vi "test_SessionManagerWrapper_StopSessionManagementService_WrapperMethodsWorkWithoutError.vi"(8 "error in":errorcluster) -> (0 "error out":errorcluster, 2 "result":string, 3 "pass":bool)   [LabVIEW 2020, in "MeasurementServerTests.lvlib" / "Session Reservation Tests.lvlib"]
uses:
  Session Reservation Tests.lvlib
  Runtime/Measurements/Measurement Plugin Session Management V1/Session Reservation/Session Reservation.lvclass
  gRPC/Generated APIs/ni/measurementlink/sessionmanagement/v1/RPC Messages/ni_measurementlink_PinMapContext.ctl
  gRPC/Generated APIs/ni/measurementlink/sessionmanagement/v1/ni.measurementlink.sessionmanagement.v1.lvlib
  gRPC/Generated APIs/ni/measurementlink/sessionmanagement/v1/RPC Messages/ni_measurementlink_sessionmanagement_v1_ReserveSessionsRequest.ctl
  Helpers/Pin Map XML Strings Global.vi
  MeasurementServerTests.lvlib
  gRPC/Generated APIs/ni/measurementlink/sessionmanagement/v1/RPC Messages/ni_measurementlink_sessionmanagement_v1_ReserveAllRegisteredSessionsRequest.ctl
  gRPC/Generated APIs/ni/measurementlink/sessionmanagement/v1/RPC Messages/ni_measurementlink_sessionmanagement_v1_ChannelMapping.ctl
  gRPC/Generated APIs/ni/measurementlink/sessionmanagement/v1/RPC Messages/nidevice_grpc_Session.ctl
  gRPC/Generated APIs/ni/measurementlink/sessionmanagement/v1/RPC Messages/ni_measurementlink_sessionmanagement_v1_SessionInformation.ctl
  gRPC/Generated APIs/ni/measurementlink/sessionmanagement/v1/RPC Messages/ni_measurementlink_sessionmanagement_v1_ReserveAllRegisteredSessionsResponse.ctl
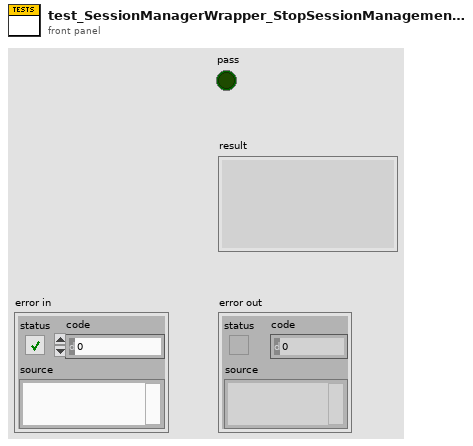
[diagram p1: front panel]
types:
  T1 = typedef "ni.measurementlink.sessionmanagement.v1.lvlib/ni_measurementlink_sessionmanagement_v1_ReserveAllRegisteredSessionsResponse.ctl" = cluster{"sessions":T2[]}
  T2 = typedef "ni.measurementlink.sessionmanagement.v1.lvlib/ni_measurementlink_sessionmanagement_v1_SessionInformation.ctl" = cluster{"session":T3, "resource_name":string, "channel_list":string, "instrument_type_id":string, "session_exists":bool, "channel_mappings":T4[]}
  T3 = typedef "ni.measurementlink.sessionmanagement.v1.lvlib/nidevice_grpc_Session.ctl" = cluster{"name":string}
  T4 = typedef "ni.measurementlink.sessionmanagement.v1.lvlib/ni_measurementlink_sessionmanagement_v1_ChannelMapping.ctl" = cluster{"pin_or_relay_name":string, "site":i32, "channel":string, "multiplexer_resource_name":string, "multiplexer_route":string}
  T5 = typedef "ni.measurementlink.sessionmanagement.v1.lvlib/ni_measurementlink_sessionmanagement_v1_ReserveAllRegisteredSessionsRequest.ctl" = cluster{"timeout_in_milliseconds":i32, "instrument_type_id":string}
  T6 = typedef "ni.measurementlink.sessionmanagement.v1.lvlib/ni_measurementlink_sessionmanagement_v1_ReserveSessionsRequest.ctl" = cluster{"pin_map_context":T7, "pin_or_relay_names":string[], "instrument_type_id":string, "timeout_in_milliseconds":i32}
  T7 = typedef "ni.measurementlink.sessionmanagement.v1.lvlib/ni_measurementlink_PinMapContext.ctl" = cluster{"pin_map_id":string, "sites":i32[]}
  T8 = typedef "ni.measurementlink.sessionmanagement.v1.lvlib/ni_measurementlink_sessionmanagement_v1_ReserveSessionsResponse.ctl" = cluster{"sessions":T2[], "multiplexer_sessions":T9[], "group_mappings":T10[]}
  T9 = typedef "ni.measurementlink.sessionmanagement.v1.lvlib/ni_measurementlink_sessionmanagement_v1_MultiplexerSessionInformation.ctl" = cluster{"session":T3, "resource_name":string, "multiplexer_type_id":string, "session_exists":bool}
  T10 = typedef "ni.measurementlink.sessionmanagement.v1.lvlib/ni_measurementlink_sessionmanagement_v1_ReserveSessionsResponse_GroupMappingsEntry.ctl" = cluster{"key":string, "value":T11}
  T11 = typedef "ni.measurementlink.sessionmanagement.v1.lvlib/ni_measurementlink_sessionmanagement_v1_ResolvedPinsOrRelays.ctl" = cluster{"pin_or_relay_names":string[]}
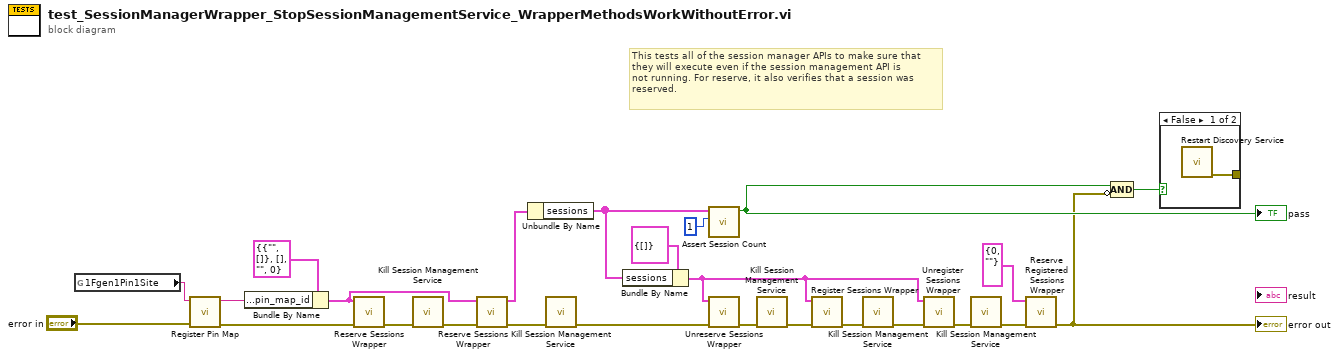
[diagram p0: block diagram]
diagram:
  # "This tests all of the session manager APIs to make sure that\nthey will execute even if the session management API is\nnot running. For reserve, it also verifies that a session was\nreserved."
  n1 = global read "Pin Map XML Strings Global.vi" "1Fgen1Pin1Site"() -> (w25:string)
  n2 = call "Register Pin Map.vi"("error in"="error in", "pin map xml"=w25) -> ("error out"=w9:errorcluster, "pin map id"=w23:string)  [unwired: 8 in]
  n3 = Bundle By Name(cluster=T6 {"pin_map_context"={"pin_map_id"="", "sites"=[]}, "pin_or_relay_names"=[], "instrument_type_id"="", "timeout_in_milliseconds"=0} ("request data"), "pin_map_context.pin_map_id"=w23) -> (w8:T6)
  n4 = call "Reserve Sessions Wrapper.vi"("error in"=w9, "request data"=w8) -> ("error out"=w6:errorcluster)  [unwired: 8 in, 1 out]
  n5 = call "Kill Session Management Service.vi"("error in"=w6) -> ("error out"=w5:errorcluster)  [unwired: 10 in]
  n6 = call "Reserve Sessions Wrapper.vi"("error in"=w5, "request data"=w8) -> ("error out"=w20:errorcluster, "response data"=w4:T8)  [unwired: 8 in]
  n7 = Unbundle By Name(w4) -> ("sessions"=w3:T2[])
  n8 = call "Kill Session Management Service.vi"("error in"=w20) -> ("error out"=w19:errorcluster)  [unwired: 10 in]
  n9 = Bundle By Name(cluster=T1 {"sessions"=[]} ("response data 2"), "sessions"=w3) -> (w1:T1)
  n10 = call "Assert Session Count.vi"("expected value"=1, "sessions infos"=w3) -> ("pass"=w12:bool)  [unwired: 8 in, 1 out]
  "pass" <- w12
  n11 = call "Unreserve Sessions Wrapper.vi"("error in"=w19, "request data"=w1) -> ("error out"=w22:errorcluster)  [unwired: 8 in, 1 out]
  n12 = call "Kill Session Management Service.vi"("error in"=w22) -> ("error out"=w18:errorcluster)  [unwired: 10 in]
  n13 = call "Register Sessions Wrapper.vi"("error in"=w18, "request data"=w1) -> ("error out"=w17:errorcluster)  [unwired: 8 in, 1 out]
  n14 = call "Kill Session Management Service.vi"("error in"=w17) -> ("error out"=w16:errorcluster)  [unwired: 10 in]
  n15 = call "Unregister Sessions Wrapper.vi"("error in"=w16, "request data"=w1) -> ("error out"=w15:errorcluster)  [unwired: 8 in, 1 out]
  n16 = call "Kill Session Management Service.vi"("error in"=w15) -> ("error out"=w14:errorcluster)  [unwired: 10 in]
  n17 = call "Reserve Registered Sessions Wrapper.vi"("error in"=w14, "request data"=T5 {"timeout_in_milliseconds"=0, "instrument_type_id"=""}) -> ("error out"=w11:errorcluster)  [unwired: 8 in, 1 out]
  "error out" <- w11
  n18 = Compound Arithmetic op=AND(w12, invert w11) -> (w21:bool)
  n19 = case shown="False" w21 {
    tunnel: [w26 _] -> _
    frame False {
      n20 = call "Restart Discovery Service.vi"() -> ("error out"=w26:errorcluster)  [unwired: 11 in]
    }
    frame True {
    }
  }
